vi "Clone Beacon.vi"(8 "error in":errorcluster) -> (0 "error out":errorcluster)   [LabVIEW 2013, in "LVTM.lvlib"]
doc: "Drop this VI into any asynchronously called reentrant VI, to force it to be seen by LabVIEW Task Manager. There is no need to drop this into a statically called reentrant VI, because these are already searched for by the tool. When the reentrant clone is created and run, it will be added to a list of clones that the tool watches. LabVIEW Task Manager will then display \"All VIs in Memory\" AND the ones added using this VI."
uses:
  LVTM.lvlib
  Clone VIs FG Enum.ctl
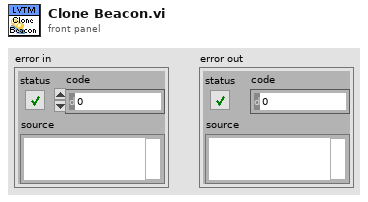
[diagram p1: front panel]
types:
  T1 = typedef "LVTM.lvlib/Clone VIs FG Enum.ctl" = enum16{"Get", "Get Active VIs", "Add VI"}
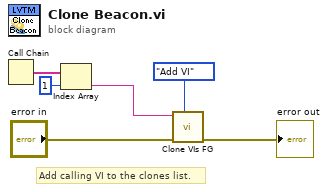
[diagram p0: block diagram]
diagram:
  # "Add calling VI to the clones list."
  n1 = Call Chain() -> (call chain=w4:string[])
  n2 = Index Array(array=w4, index=1) -> (element=w2:string)
  n3 = call "Clone VIs FG.vi"("Action (Add VI)"=Clone_VIs_FG_Enum."Add VI", "error in"="error in", "VI Name"=w2) -> ("error out"=→"error out":errorcluster)  [unwired: 7 in, 1 out]
